vi "week03_Ex1.vi"() -> ()   [LabVIEW 2017]
panel:
  out "s? t:f":string
  out "x = 0?":bool
  out "Conuter":i16
  in  "IN 1":bool
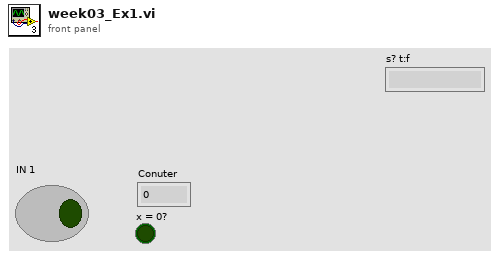
[diagram p1: front panel]
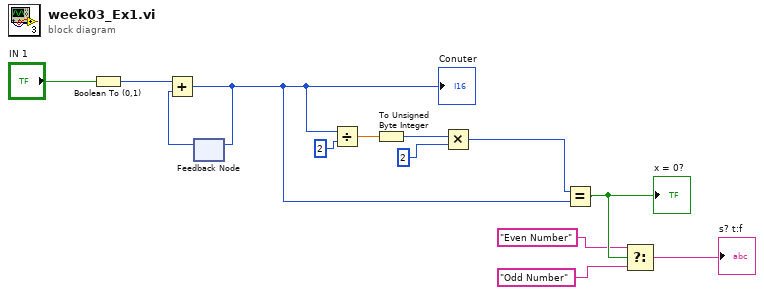
[diagram p0: block diagram]
diagram:
  n1 = Boolean To (0,1)(Boolean="IN 1") -> (0, 1=w12:i16)
  n2 = feedback #1() -> (w11:i16)  [unwired: 1 in]
  n3 = Add(x=w12, y=w11) -> (x+y=w5:i16)
  "Conuter" <- w5
  n4 = feedback-in #1(w5) -> ()
  n5 = Divide(x=w5, y=2) -> (x/y=w9:dbl)
  n6 = To Unsigned Byte Integer(number=w9) -> (unsigned 8bit integer=w8:u8)
  n7 = Multiply(x=w8, y=2) -> (x*y=w6:i32)
  n8 = Equal?(x=w6, y=w5) -> (x = y?=w4:bool)
  "x = 0?" <- w4
  n9 = Select(t="Even Number", s=w4, f="Odd Number") -> (s? t:f=→"s? t:f":string)
